vi "Symphony DatSock_Write.vi"() -> ()   [LabVIEW 2019]
panel:
  in  "stop":bool
  in  "Write":bool
  out "Tableau":dbl[][](array[numeric])
  in  "DIm1 Col":i32
  in  "DIm1 Row":i32
  in  "URL":string
  in  "entrée d'erreur (pas d'erreur)":errorcluster
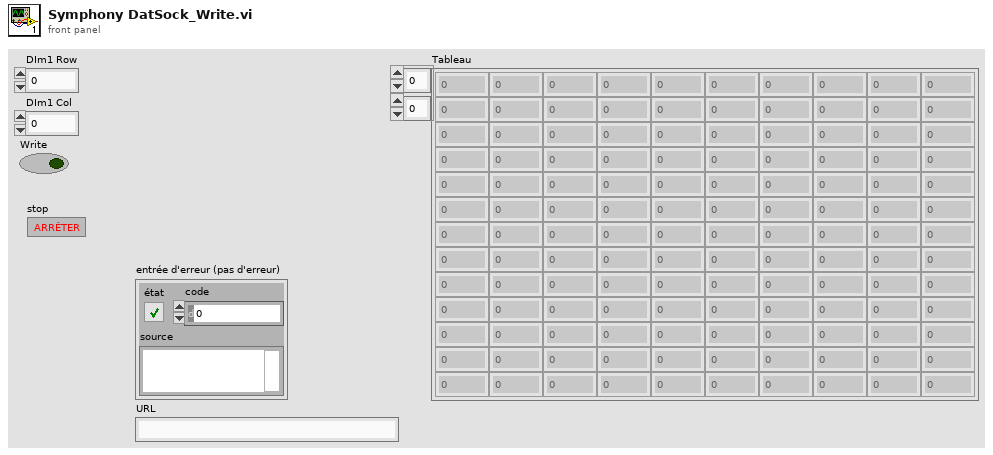
[diagram p1: front panel]
types:
  T1 = enum16{"Read", "Write", "ReadWrite", "BufferedRead", "BufferedReadWrite"}
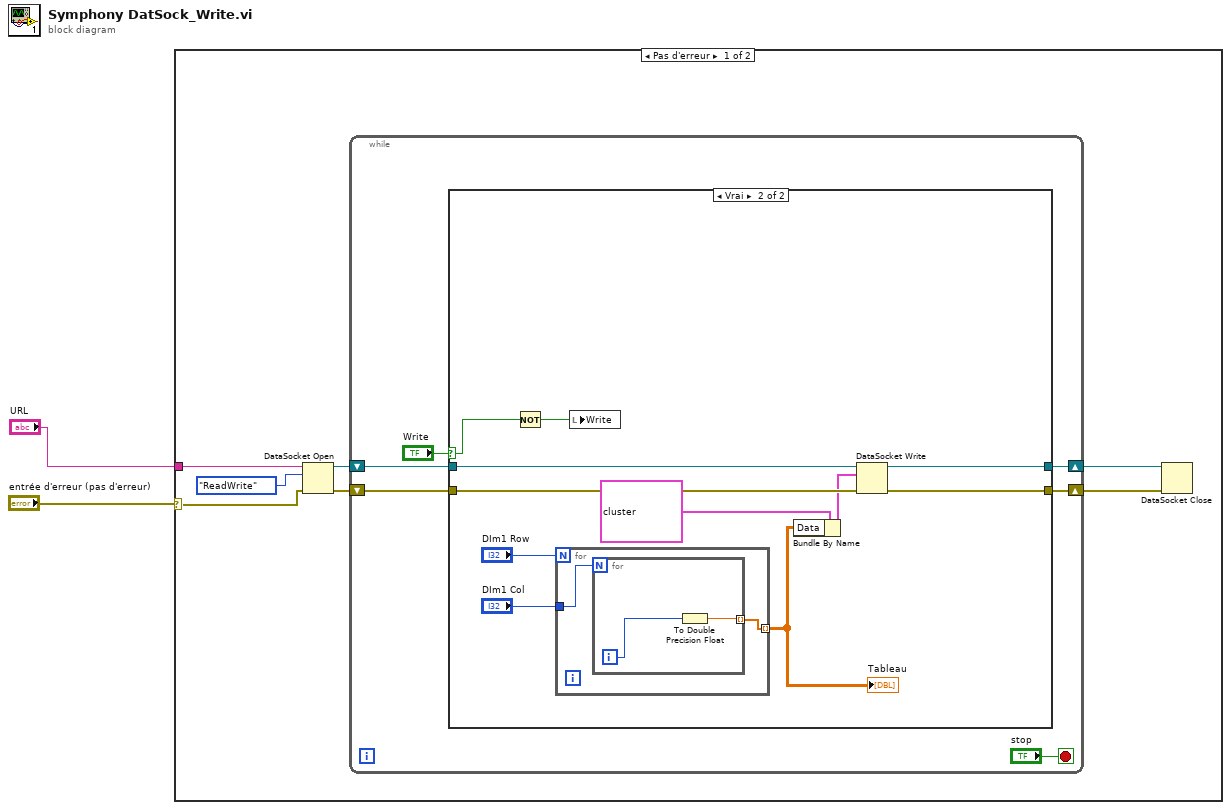
[diagram p0: block diagram]
diagram:
  n1 = case shown="Pas d'erreur" "entrée d'erreur (pas d'erreur)" {
    selector: "entrée d'erreur (pas d'erreur)" -> [w8 _]
    tunnel: "URL" -> [w9 _]
    frame No Error {
      n2 = DataSocket Open(8:w8, 10:T1."ReadWrite" ("mode"), 11:w9) -> (0:w6:errorcluster, 3:w5:refnum<k13>)  [unwired: 1 in]
      n3 = while {
        shift-right: [w13] -> w4
        shift-left: w6 -> [w15]
        shift-right: [w12] -> w3
        shift-left: w5 -> [w14]
        stop <- "stop" stop-if-true
        n4 = case shown="Vrai" "Write" {
          selector: "Write" -> [_ w19]
          tunnel: w15 -> [w17 w28]
          tunnel: w14 -> [w16 w27]
          tunnel: [w17 w23] -> w13
          tunnel: [w16 w22] -> w12
          frame False {
          }
          frame True {
            n5 = Not(x=w19) -> (.not. x?=w18:bool)
            n6 = for {
              N: "DIm1 Row" -> [_]
              tunnel: [w30] -> w24 mode=indexing
              tunnel: "DIm1 Col" -> [w29]
              n7 = for {
                N: w29 -> [_]
                tunnel: [w32] -> w30 mode=indexing
                i -> [w31]
                n8 = To Double Precision Float(number=w31) -> (double precision float=w32:dbl)
              }
            }
            "Tableau" <- w24
            n9 = local write "Write"(w18) -> ()
            n10 = Bundle By Name(cluster=cluster{"Message":string, "Data":variant, i32} {"Message"="test message", "Data"=variant, 0} ("élément"), "Data"=w24) -> (w25:cluster{"Message":string, "Data":variant, i32})
            n11 = DataSocket Write(8:w28, 10:w25, 11:w27) -> (0:w23:errorcluster, 3:w22:refnum<k13>)  [unwired: 1 in, 1 out]
          }
        }
      }
      n12 = DataSocket Close(8:w4, 11:w3) -> ()  [unwired: 1 in, 2 out]
    }
    frame Error {
    }
  }
